vi "myfgvtimer.vi"() -> ()   [LabVIEW 2018]
panel:
  out "pause flag":bool
  in  "Enum":enum16{"init", "reset", "pause", "run"}(ring)=enum."reset"
  out "x-y":dbl
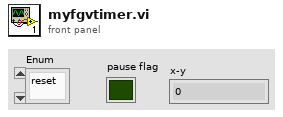
[diagram p1: front panel]
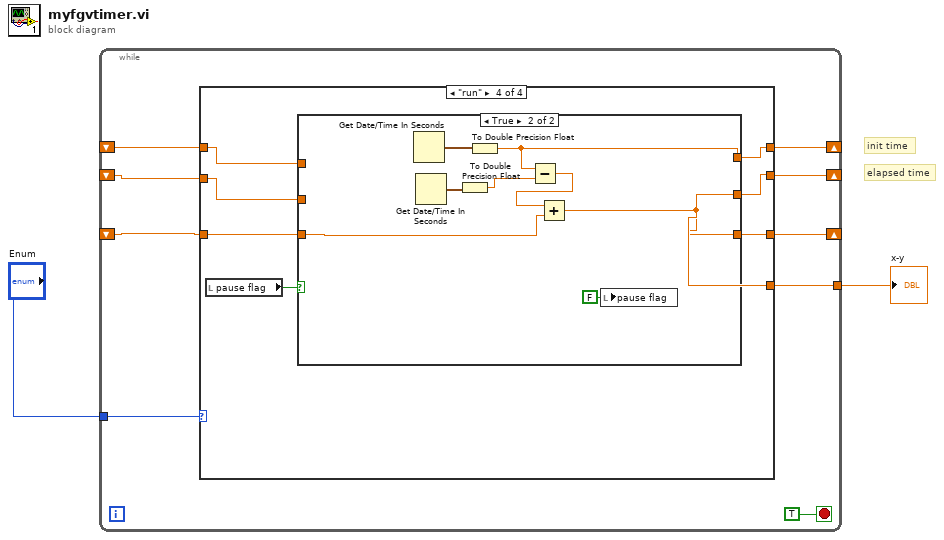
[diagram p0: block diagram]
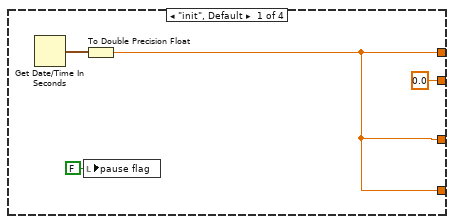
[diagram p2: hidden frame]
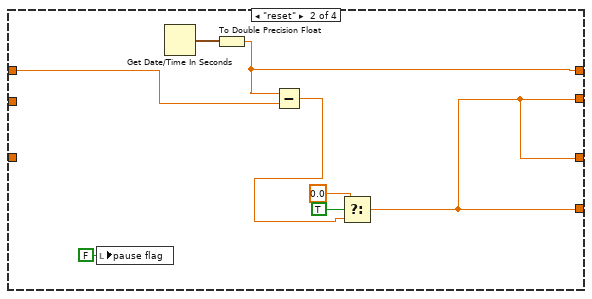
[diagram p3: hidden frame]
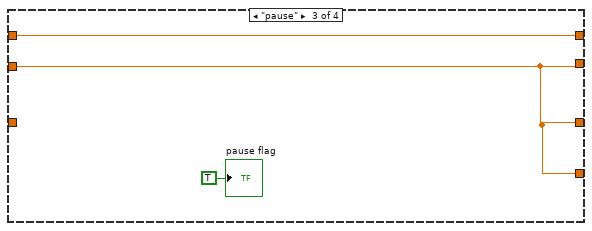
[diagram p4: hidden frame]
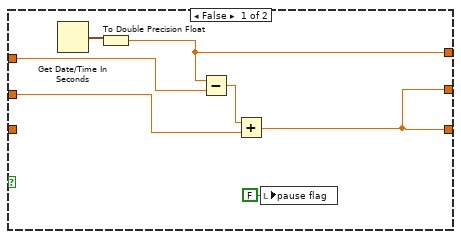
[diagram p5: hidden frame]
diagram:
  # "elapsed time"
  # "init time"
  n1 = while {
    tunnel: "Enum" -> [w11]
    shift-right: [w10] -> _
    shift-left: _ -> [w9]
    tunnel: [w7] -> w1
    shift-right: [w6] -> _
    shift-left: _ -> [w5]
    shift-right: [w4] -> _
    shift-left: _ -> [w3]
    stop <- TRUE stop-if-true
    n2 = case shown="\"run\"" w11 {
      tunnel: [w12 w16 w24 w30] -> w10
      tunnel: w9 -> [_ w22 w24 w33]
      tunnel: [w12 w17 w25 w31] -> w7
      tunnel: [0.0 w17 w25 w31] -> w6
      tunnel: w5 -> [_ _ w25 w32]
      tunnel: [w12 w17 w25 w27] -> w4
      tunnel: w3 -> [_ _ _ w28]
      frame "init", Default {
        n3 = Get Date/Time In Seconds() -> (seconds since 1Jan1904=w15:timestamp)
        n4 = local write "pause flag"(FALSE ("Boolean")) -> ()
        n5 = To Double Precision Float(number=w15) -> (double precision float=w12:dbl)
      }
      frame "reset" {
        n6 = local write "pause flag"(FALSE ("Boolean")) -> ()
        n7 = Get Date/Time In Seconds() -> (seconds since 1Jan1904=w23:timestamp)
        n8 = To Double Precision Float(number=w23) -> (double precision float=w16:dbl)
        n9 = Subtract(x=w16, y=w22) -> (x-y=w19:dbl)
        n10 = Select(t=0.0, s=TRUE, f=w19) -> (s? t:f=w17:dbl)
      }
      frame "pause" {
        "pause flag" <- TRUE ("Boolean")
      }
      frame "run" {
        n11 = local read "pause flag"() -> (w29:bool)
        n12 = case shown="True" w29 {
          tunnel: w33 -> [w39 _]
          tunnel: w32 -> [w37 _]
          tunnel: [w35 w43] -> w31
          tunnel: [w36 w45] -> w30
          tunnel: w28 -> [_ w47]
          tunnel: [w35 w43] -> w27
          frame False {
            n13 = Get Date/Time In Seconds() -> (seconds since 1Jan1904=w40:timestamp)
            n14 = To Double Precision Float(number=w40) -> (double precision float=w36:dbl)
            n15 = Subtract(x=w36, y=w39) -> (x-y=w38:dbl)
            n16 = Add(x=w38, y=w37) -> (x+y=w35:dbl)
            n17 = local write "pause flag"(FALSE ("Boolean")) -> ()
          }
          frame True {
            n18 = Get Date/Time In Seconds() -> (seconds since 1Jan1904=w46:timestamp)
            n19 = Get Date/Time In Seconds() -> (seconds since 1Jan1904=w42:timestamp)
            n20 = To Double Precision Float(number=w42) -> (double precision float=w41:dbl)
            n21 = To Double Precision Float(number=w46) -> (double precision float=w45:dbl)
            n22 = Subtract(x=w45, y=w41) -> (x-y=w44:dbl)
            n23 = Add(x=w44, y=w47) -> (x+y=w43:dbl)
            n24 = local write "pause flag"(FALSE ("Boolean")) -> ()
          }
        }
      }
    }
  }
  "x-y" <- w1
